vi "Test-DeviceCMD.vi"(7 "DeviceData":T1) -> ()   [LabVIEW 2020]
panel:
  out "Boolean":bool
  out "Name":string
  out "CMD":T2
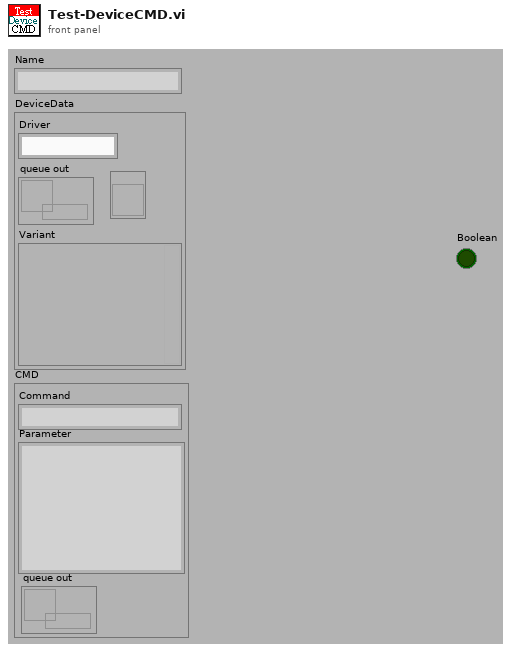
[diagram p1: front panel]
types:
  T1 = cluster{"Driver":string, "queue out":refnum<queue>, refnum<vi>, "Variant":variant}
  T2 = cluster{"Command":string, "Parameter":string, "queue out":refnum<queue>}
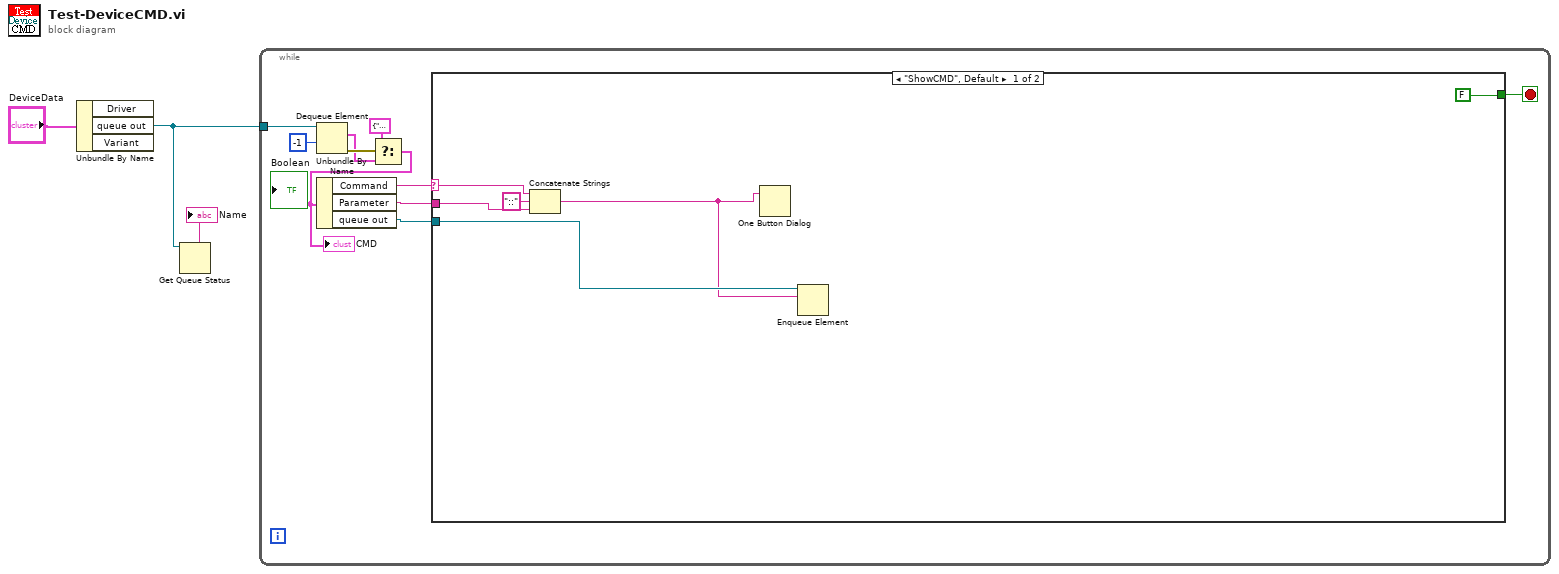
[diagram p0: block diagram]
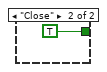
[diagram p2: hidden frame]
diagram:
  n1 = Unbundle By Name("DeviceData") -> ("queue out"=w2:refnum<queue>)  [unwired: 2 out]
  n2 = Get Queue Status(queue=w2) -> (queue name=→"Name":string)  [unwired: 2 in, 7 out]
  n3 = while {
    tunnel: w2 -> [w13]
    stop <- w9 stop-if-true
    n4 = Dequeue Element(queue=w13, timeout in ms (-1)=-1) -> (element=w6:T2, error out=w7:errorcluster)  [unwired: 1 in, 2 out]
    n5 = Select(t=T2 {"Command"="Close", "Parameter"="", "queue out"=refnum}, s=w7, f=w6) -> (s? t:f=w5:T2)
    "CMD" <- w5
    n6 = Unbundle By Name(w5) -> ("Command"=w12:string, "Parameter"=w11:string, "queue out"=w10:refnum<queue>)
    n7 = case shown="\"ShowCMD\", Default" w12 {
      selector: w12 -> [w18 _]
      tunnel: w11 -> [w17 _]
      tunnel: w10 -> [w15 _]
      tunnel: [FALSE TRUE] -> w9
      frame "ShowCMD", Default {
        n8 = Concatenate Strings(w18, "::" ("string"), w17) -> (w14:string)
        n9 = One Button Dialog(message=w14) -> ()  [unwired: 1 in, 1 out]
        n10 = Enqueue Element(queue=w15, element=w14) -> ()  [unwired: 2 in, 3 out]
      }
      frame "Close" {
      }
    }
  }
